vi "SinusBessel.vi"(2 "Amplitude A":dbl=1.0, 3 "Bessel v":dbl=1.0, 4 "Zahl der Punkte N":dbl=1000.0, 5 "Phase phi":dbl=1.0, 6 "Frequenz f":dbl=1.0) -> (0 "y":dbl[](array[numeric]), 1 "Zeit t":dbl[](array[numeric]))   [LabVIEW 2017]
doc: "Sinusundbessel"
uses:
  <vilib>/gmath/NI_Gmath.lvlib
panel:
  out "Bessel":cluster{"Y":dbl[], "Y":dbl[]}[](graph)
  out "Sinus":cluster{"Y":dbl[], "Y":dbl[]}[](graph)
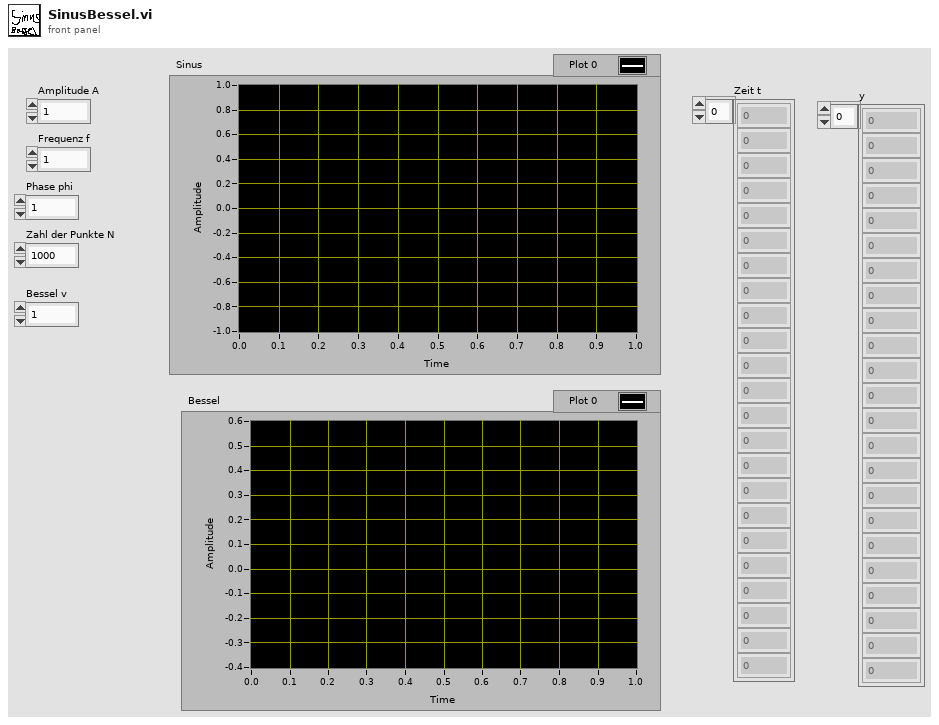
[diagram p1: front panel]
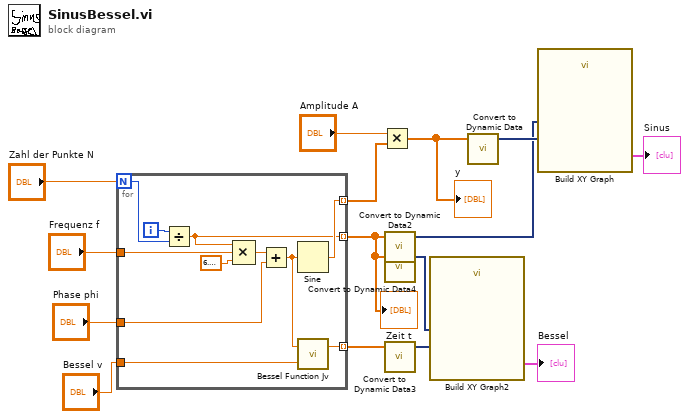
[diagram p0: block diagram]
diagram:
  n1 = for {
    N: "Zahl der Punkte N" -> [w26]
    tunnel: "Frequenz f" -> [w24]
    tunnel: "Phase phi" -> [w21]
    tunnel: [w20] -> w2 mode=indexing
    tunnel: [w19] -> w4 mode=indexing
    tunnel: "Bessel v" -> [w17]
    tunnel: [w16] -> w6 mode=indexing
    i -> [w25]
    n2 = Divide(x=w25, y=w26) -> (x/y=w19:dbl)
    n3 = Compound Arithmetic op=MULTIPLY(w19, w24, 6.283185307179586) -> (w22:dbl)
    n4 = Add(x=w22, y=w21) -> (x+y=w18:dbl)
    n5 = Sine(x=w18) -> (sin(x)=w20:dbl)
    n6 = call <vilib>:"Bessel Function Jv.vi"("v"=w17, "x"=w18) -> ("Jv(x)"=w16:dbl)  [unwired: 1 in]
  }
  "Zeit t" <- w4
  n7 = Multiply(x="Amplitude A", y=w2) -> (x*y=w1:dbl[])
  "y" <- w1
  n8 = call "Convert to Dynamic Data2"("Array"=w4) -> ("Dynamic Data Type"=w9:dynamicdata)  [unwired: 3 in]
  n9 = call "Convert to Dynamic Data4"("Array"=w4) -> ("Dynamic Data Type"=w3:dynamicdata)  [unwired: 3 in]
  n10 = call "Convert to Dynamic Data3"("Array"=w6) -> ("Dynamic Data Type"=w5:dynamicdata)  [unwired: 3 in]
  n11 = call "Build XY Graph2"("Y Input"=w5, "X Input"=w3) -> ("XY Graph"=→"Bessel":cluster{"X":dbl[], "Y":dbl[]}[])  [unwired: 8 in, 1 out]
  n12 = call "Convert to Dynamic Data"("Array"=w1) -> ("Dynamic Data Type"=w10:dynamicdata)  [unwired: 3 in]
  n13 = call "Build XY Graph"("Y Input"=w10, "X Input"=w9) -> ("XY Graph"=→"Sinus":cluster{"X":dbl[], "Y":dbl[]}[])  [unwired: 8 in, 1 out]
